vi "Get Node Info.vi"(8 "error in (no error)":errorcluster, 11 "Vecto in":refnum<class "Vecto.lvclass">) -> (0 "error out":errorcluster, 2 "Info":T1, 3 "Vecto out":refnum<class "Vecto.lvclass">)   [LabVIEW 2020, in "Vecto.lvlib" / "Vecto.lvclass"]
uses:
  Vecto.lvclass
  Vecto.lvclass/Vecto.ctl
  Node Config/Node Config.lvclass
  Node Config/Node Info.ctl
  VectoConfig/VectoConfig.lvlib
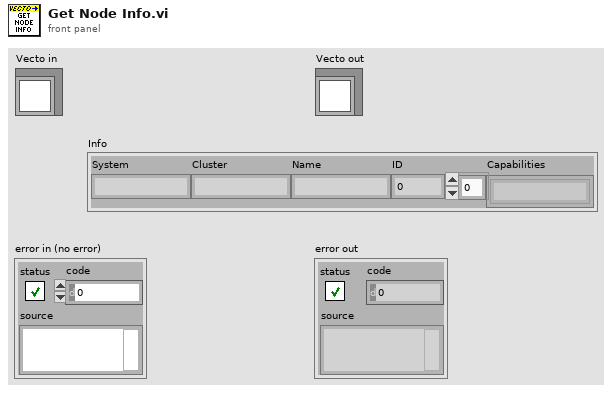
[diagram p1: front panel]
types:
  T1 = typedef "VectoConfig.lvlib/Node Info.ctl" = cluster{"System":string, "Cluster":string, "Name":string, "ID":u32, "Capabilities":string[]}
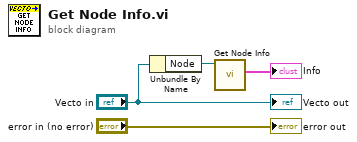
[diagram p0: block diagram]
diagram:
  n1 = Unbundle By Name("Vecto in") -> ("Node"=w2:refnum<class "Node Config.lvclass">)
  n2 = call "Get Node Info.vi"("Node Config in"=w2) -> ("Info"=→"Info":T1)  [unwired: 8 in, 2 out]
  "error out" <- "error in (no error)"
  "Vecto out" <- "Vecto in"
